vi "Next Page.vi"(8 "error in (no error)":errorcluster, 11 "Sensor Model in":refnum<class "Sensor Model.lvclass">) -> (0 "error out":errorcluster, 3 "Sensor Model out":refnum<class "Sensor Model.lvclass">)   [LabVIEW 2013, in "Sensor Model.lvlib" / "Sensor Model.lvclass"]
uses:
  Sensor Model.lvclass
  Sensor Model.lvclass/Sensor Model.ctl
  <vilib>/ActorFrameworkMVC/View Observer/View Registry/View Registry.lvclass/View Registry.ctl
  Sensor Model Messages/Abstract Sensor Move In Next Msg/Abstract Sensor Move In Next Msg.lvclass
  <vilib>/ActorFrameworkMVC/View Observer/View Registry/View Registry.lvclass
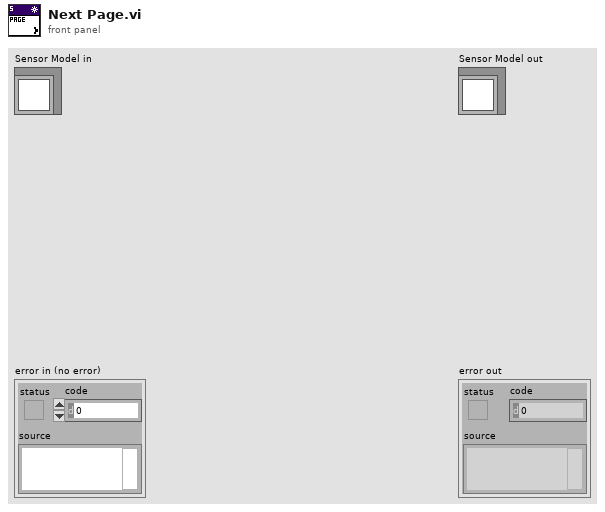
[diagram p1: front panel]
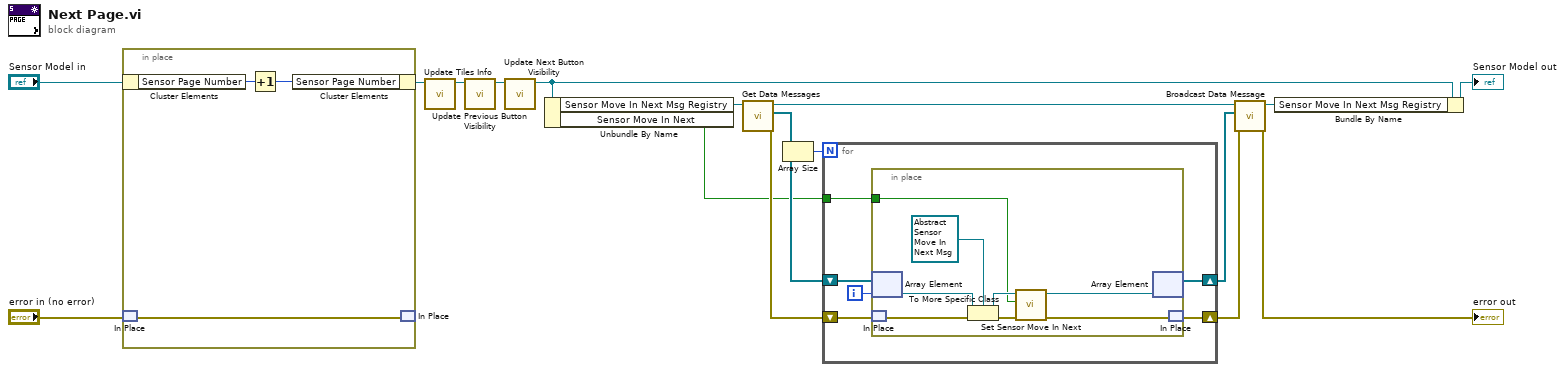
[diagram p0: block diagram]
diagram:
  n1 = in-place {
    n2 = in-place-cluster #1("Sensor Model in") -> ("Sensor Page Number"=w20:i32)
    n3 = in-place-match #2("error in (no error)") -> (w18:errorcluster)
    n4 = Increment(x=w20) -> (x+1=w19:i32)
    n5 = in-place-cluster #1("Sensor Page Number"=w19) -> (w6:refnum<class "Sensor Model.lvclass">)
    n6 = in-place-match #2(w18) -> ()  [unwired: 1 out]
  }
  n7 = call "Update Tiles Info.vi"("Sensor Model in"=w6) -> ("Sensor Model out"=w5:refnum<class "Sensor Model.lvclass">)  [unwired: 9 in, 1 out]
  n8 = call "Update Previous Button Visibility.vi"("Sensor Model in"=w5) -> ("Sensor Model out"=w4:refnum<class "Sensor Model.lvclass">)  [unwired: 9 in, 1 out]
  n9 = call "Update Next Button Visibility.vi"("Sensor Model in"=w4) -> ("Sensor Model out"=w3:refnum<class "Sensor Model.lvclass">)  [unwired: 9 in, 1 out]
  n10 = Unbundle By Name(w3) -> ("Sensor Move In Next Msg Registry"=w2:refnum<class "View Registry.lvclass">, "Sensor Move In Next"=w9:bool)
  n11 = call <vilib>:"Get Data Messages.vi"("View Registry in"=w2) -> ("error out"=w13:errorcluster, "Data Messages"=w14:refnum<class "Data Message.lvclass">[], "View Registry out"=w1:refnum<class "View Registry.lvclass">)  [unwired: 8 in]
  n12 = Array Size(array=w14) -> (size(s)=w15:i32)
  n13 = for {
    N: w15 -> [_]
    shift-right: [w25] -> w12
    shift-left: w14 -> [w26]
    shift-right: [w22] -> w11
    shift-left: w13 -> [w24]
    tunnel: w9 -> [w23]
    i -> [w21]
    n14 = in-place {
      in-place-border: w23 -> [w27]
      n15 = in-place-array #3(w26, w21) -> (w32:refnum<class "Data Message.lvclass">)
      n16 = in-place-match #4(w24) -> (w34:errorcluster)
      n17 = To More Specific Class(target class=refnum<class "Abstract Sensor Move In Next Msg.lvclass"> refnum ("Sensor Model.lvlib:Abstract Sensor Move In Next Msg.lvclass"), reference=w32, error in=w34) -> (specific class reference=w28:refnum<class "Abstract Sensor Move In Next Msg.lvclass">, error out=w31:errorcluster)
      n18 = call "Set Sensor Move In Next.vi"("error in (no error)"=w31, "Sensor Move In Next"=w27, "Abstract Sensor Move In Next Msg in"=w28) -> ("error out"=w30:errorcluster, "Abstract Sensor Move In Next Msg out"=w29:refnum<class "Abstract Sensor Move In Next Msg.lvclass">)  [unwired: 7 in]
      n19 = in-place-array #3(w29) -> (w25:refnum<class "Data Message.lvclass">[])  [unwired: 1 out]
      n20 = in-place-match #4(w30) -> (w22:errorcluster)
    }
  }
  n21 = call <vilib>:"Broadcast Data Message.vi"("error in (no error)"=w11, "Data Messages"=w12, "View Registry in"=w1) -> ("error out"=→"error out":errorcluster, "View Registry out"=w10:refnum<class "View Registry.lvclass">)  [unwired: 7 in]
  n22 = Bundle By Name(cluster=w3, "Sensor Move In Next Msg Registry"=w10) -> (→"Sensor Model out":refnum<class "Sensor Model.lvclass">)
